vi "Q.Ping.vi"(7 "Target Q Name":string, 8 "Error In":errorcluster, 10 "Timeout(ms)":i32=100, 11 "Target Q In":refnum<queue>) -> (0 "Error Out":errorcluster, 1 "Success":bool, 2 "Latency(s)":dbl, 3 "Target Q Out":refnum<queue>)   [LabVIEW 2024, in "EQMF.lvlib" / "Queue Utils.lvlib"]
doc: "This VI enqueues an element to the Queue.\nIf the 'Q Name' input is not empty then it obtains the queue by name.\n If a queue is ontained by name and this queue does nto already exits, an error is generated.\nIf the 'Q Name' input is empty then it uses the 'Q In' for obtaining the queue.\n\nBy default the 'Top of Q' input is FALSE to put this element on bottom of the queue.\nSet 'Top of Q' to TRUE to enqueue this command at the top of the queue."
uses:
  Queue Utils.lvlib
  Q.Element.ctl
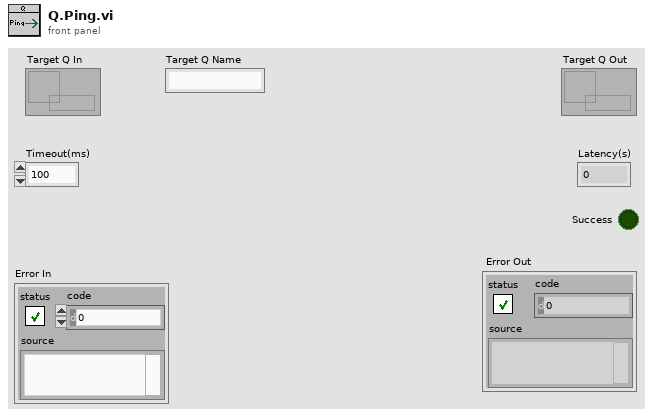
[diagram p1: front panel]
types:
  T1 = typedef "EQMF.lvlib/Queue Utils.lvlib/Q.Element.ctl" = cluster{"Cmd":string, "Sub":string, "Data1":variant, "Data2":variant}
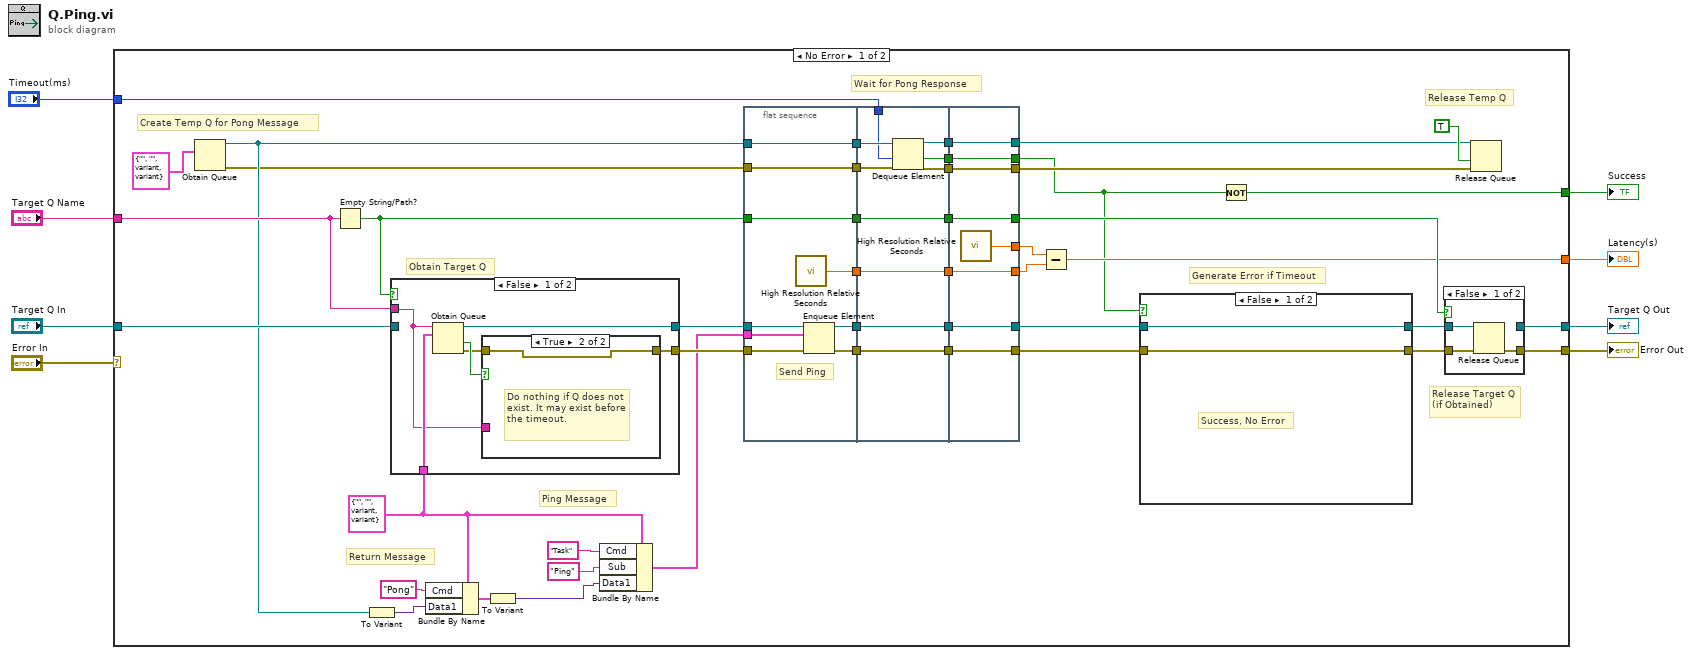
[diagram p0: block diagram]
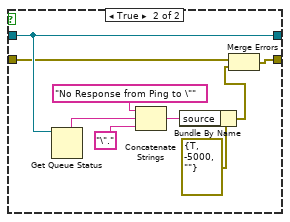
[diagram p2: hidden frame]
diagram:
  n1 = case shown="No Error" "Error In" {
    selector: "Error In" -> [_ w107]
    tunnel: [w15 w107] -> w8
    tunnel: "Target Q Name" -> [w52 _]
    tunnel: "Target Q In" -> [w53 w106]
    tunnel: [w51 w106] -> w4
    tunnel: "Timeout(ms)" -> [w35 _]
    tunnel: [w20 _] -> w2
    tunnel: [w9 _] -> w1
    frame No Error {
      w43 = T1 {"Cmd"="", "Sub"="", "Data1"=variant, "Data2"=variant}
      # "Generate Error if Timeout"
      # "Release Target Q\n(if Obtained)"
      # "Wait for Pong Response"
      # "Release Temp Q"
      # "Ping Message"
      # "Return Message"
      # "Create Temp Q for Pong Message"
      # "Obtain Target Q"
      n2 = Obtain Queue(element data type=T1 {"Cmd"="", "Sub"="", "Data1"=variant, "Data2"=variant}) -> (queue out=w41:refnum<queue>, error out=w38:errorcluster)  [unwired: 4 in, 1 out]
      n3 = Empty String/Path?(string/path=w52) -> (empty?=w37:bool)
      n4 = To Variant(anything=w41) -> (Variant=w46:variant)
      n5 = case shown="False" w37 {
        tunnel: [w97 _] -> w18
        tunnel: [w102 w105] -> w19
        tunnel: w52 -> [w98 _]
        tunnel: w43 -> [w101 _]
        tunnel: w53 -> [_ w105]
        frame False {
          n6 = Obtain Queue(name (unnamed)=w98, element data type=w101) -> (queue out=w102:refnum<queue>, created new?=w100:bool, error out=w99:errorcluster)  [unwired: 3 in]
          n7 = case shown="True" w100 {
            tunnel: w99 -> [w103 w104]
            tunnel: w98 -> [_ _]
            tunnel: [w103 w104] -> w97
            frame False {
            }
            frame True {
              # "Do nothing if Q does not exist. It may exist before the timeout."
            }
          }
        }
        frame True {
        }
      }
      n8 = Bundle By Name(cluster=w43, "Cmd"="Pong", "Data1"=w46) -> (w45:T1)
      n9 = To Variant(anything=w45) -> (Variant=w44:variant)
      n10 = Bundle By Name(cluster=w43, "Cmd"="Task", "Sub"="Ping" ("Cmd"), "Data1"=w44) -> (w17:T1)
      n11 = flat-sequence {
        tunnel: w37 -> [w71]
        tunnel: w18 -> [w67]
        tunnel: w19 -> [w68]
        tunnel: w38 -> [w72]
        tunnel: w41 -> [w73]
        tunnel: [w73] -> w34
        tunnel: [w72] -> w33
        tunnel: [w66] -> w32
        tunnel: [w71] -> w31
        tunnel: [w70] -> w25
        tunnel: w17 -> [w69]
        tunnel: [w65] -> w16
        tunnel: w35 -> [w76]
        tunnel: w34 -> [w83]
        tunnel: w33 -> [w80]
        tunnel: w32 -> [w78]
        tunnel: w31 -> [w77]
        tunnel: [w82] -> w30
        tunnel: [w81] -> w29
        tunnel: [w79] -> w28
        tunnel: [w78] -> w27
        tunnel: [w77] -> w26
        tunnel: w25 -> [w75]
        tunnel: [w75] -> w24
        tunnel: [w74] -> w23
        tunnel: w16 -> [w79]
        tunnel: [w87] -> w36
        tunnel: [w88] -> w13
        tunnel: [w89] -> w14
        tunnel: [w90] -> w39
        tunnel: [w91] -> w40
        tunnel: w30 -> [w91]
        tunnel: w29 -> [w90]
        tunnel: w28 -> [w89]
        tunnel: w27 -> [w88]
        tunnel: w26 -> [w87]
        tunnel: [w86] -> w21
        tunnel: w24 -> [w85]
        tunnel: [w85] -> w22
        tunnel: w23 -> [w84]
        tunnel: [w84] -> w10
        frame #0 {
          # "Send Ping"
          n12 = call <vilib>:"High Resolution Relative Seconds.vi"() -> ("relative seconds"=w70:dbl)
          n13 = Enqueue Element(queue=w68, element=w69, error in (no error)=w67) -> (queue out=w65:refnum<queue>, error out=w66:errorcluster)  [unwired: 1 in, 1 out]
        }
        frame #1 {
          n14 = Dequeue Element(queue=w83, timeout in ms (-1)=w76, error in (no error)=w80) -> (queue out=w82:refnum<queue>, timed out?=w74:bool, error out=w81:errorcluster)  [unwired: 1 out]
        }
        frame #2 {
          n15 = call <vilib>:"High Resolution Relative Seconds.vi"() -> ("relative seconds"=w86:dbl)
        }
      }
      n16 = Subtract(x=w21, y=w22) -> (x-y=w20:dbl)
      n17 = case shown="False" w10 {
        tunnel: w14 -> [w54 w59]
        tunnel: w13 -> [w55 w58]
        tunnel: [w54 w59] -> w12
        tunnel: [w55 w57] -> w11
        frame False {
          # "Success, No Error"
        }
        frame True {
          n18 = Get Queue Status(queue=w59) -> (queue name=w64:string)  [unwired: 2 in, 7 out]
          n19 = Concatenate Strings("No Response from Ping to \"", w64, "\".") -> (w60:string)
          n20 = Bundle By Name(cluster=errorcluster {"status"=TRUE, "code"=-5000, "source"=""} ("error constant"), "source"=w60) -> (w56:errorcluster)
          n21 = Merge Errors(w58, w56) -> (w57:errorcluster)
        }
      }
      n22 = Not(x=w10) -> (.not. x?=w9:bool)
      n23 = case shown="False" w36 {
        tunnel: [w94 w96] -> w15
        tunnel: w12 -> [w93 w95]
        tunnel: w11 -> [w92 w96]
        tunnel: [_ w95] -> w51
        frame False {
          n24 = Release Queue(queue=w93, error in (no error)=w92) -> (error out=w94:errorcluster)  [unwired: 1 in, 2 out]
        }
        frame True {
        }
      }
      n25 = Release Queue(queue=w40, force destroy? (F)=TRUE, error in (no error)=w39) -> ()  [unwired: 3 out]
    }
    frame Error {
    }
  }
  "Error Out" <- w8
  "Target Q Out" <- w4
  "Latency(s)" <- w2
  "Success" <- w1
